vi "LDA_CALCULATOR.vi"() -> ()   [LabVIEW 2013]
uses:
  <vilib>/Utility/file.llb/Read From Spreadsheet File (string).vi
  <vilib>/Utility/file.llb/Read From Spreadsheet File (I64).vi
  <vilib>/Utility/file.llb/Read From Spreadsheet File (DBL).vi
  <vilib>/Analysis/Matrix/Numeric/Conversions/Matrix To Array - RM.vi
  <vilib>/Utility/file.llb/Write To Spreadsheet File (DBL).vi
  <vilib>/Utility/file.llb/Write To Spreadsheet File (I64).vi
  <vilib>/Analysis/Matrix/NI_Matrix.lvlib
panel:
  in  "피험자 이름":path
  in  "SVM_SWLDA_filename":string="SVM_SWLDA_MODEL"
  in  "svm_parameter":T1={"svm_type"=0, "kernel_type"=3, "degree"=3, "gamma"=0.07, "coef0"=0.0, "cache_size"=100.0, "epsilon"=0.001, "C"=1.0, "nr_weight"=0, "weight_label"=[1, 12], "Weight (C(class i))"=[1.0, 1.0], "nu"=0.5, "p"=0.1, "Shrinking"=1, "probability"=1} {"p" format="%.4f"; "nu" format="%.4f"; "Weight (C(class i))" format="%.2f"; "C" format="%.2f"; "epsilon" format="%.4f"; "cache_size" format="%.2f"; "coef0" format="%.2f"; "gamma" format="%.5f"; "kernel_type" items=["Linear", "Poly", "RBF", "Sigmoid"]; "svm_type" items=["C-SVC", "Nu-SVC", "One-class SVM", "epsilon-SVR", "nu-SVR"]}
  in  "SVMfilename":string="SVM_MODEL"
  in  "SWLDA_PREMOVE":dbl=0.1
  in  "SWLDA_PENTER":dbl=0.05
  out "Nontarget_order_array":i64[][](array[numeric])
  out "Target_order_array":i64[](array[numeric])
  out "error out":errorcluster={"status"=TRUE, "code"=10, "source"="Create Folder in Trainging_Set_For_ LDA_Matrix_RSVP.vi<APPEND>\nC:\\Emotion_Research\\_Training_Test(LDA)\\2014-08-30"}
  # "INPUTS"
  # "SWLDA"
  # "SVM"
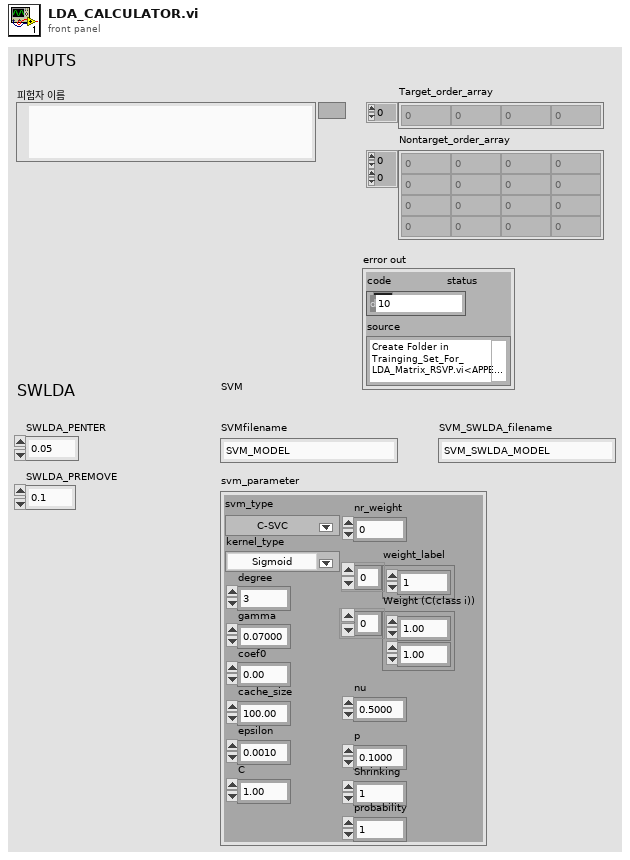
[diagram p1: front panel]
types:
  T1 = cluster{"svm_type":i16, "kernel_type":i16, "degree":i16, "gamma":dbl, "coef0":dbl, "cache_size":dbl, "epsilon":dbl, "C":dbl, "nr_weight":i16, "weight_label":i16[], "Weight (C(class i))":dbl[], "nu":dbl, "p":dbl, "Shrinking":i16, "probability":i16}
  T2 = typedef "NI_Matrix.lvlib/RealMatrix.ctl" = dbl[][]
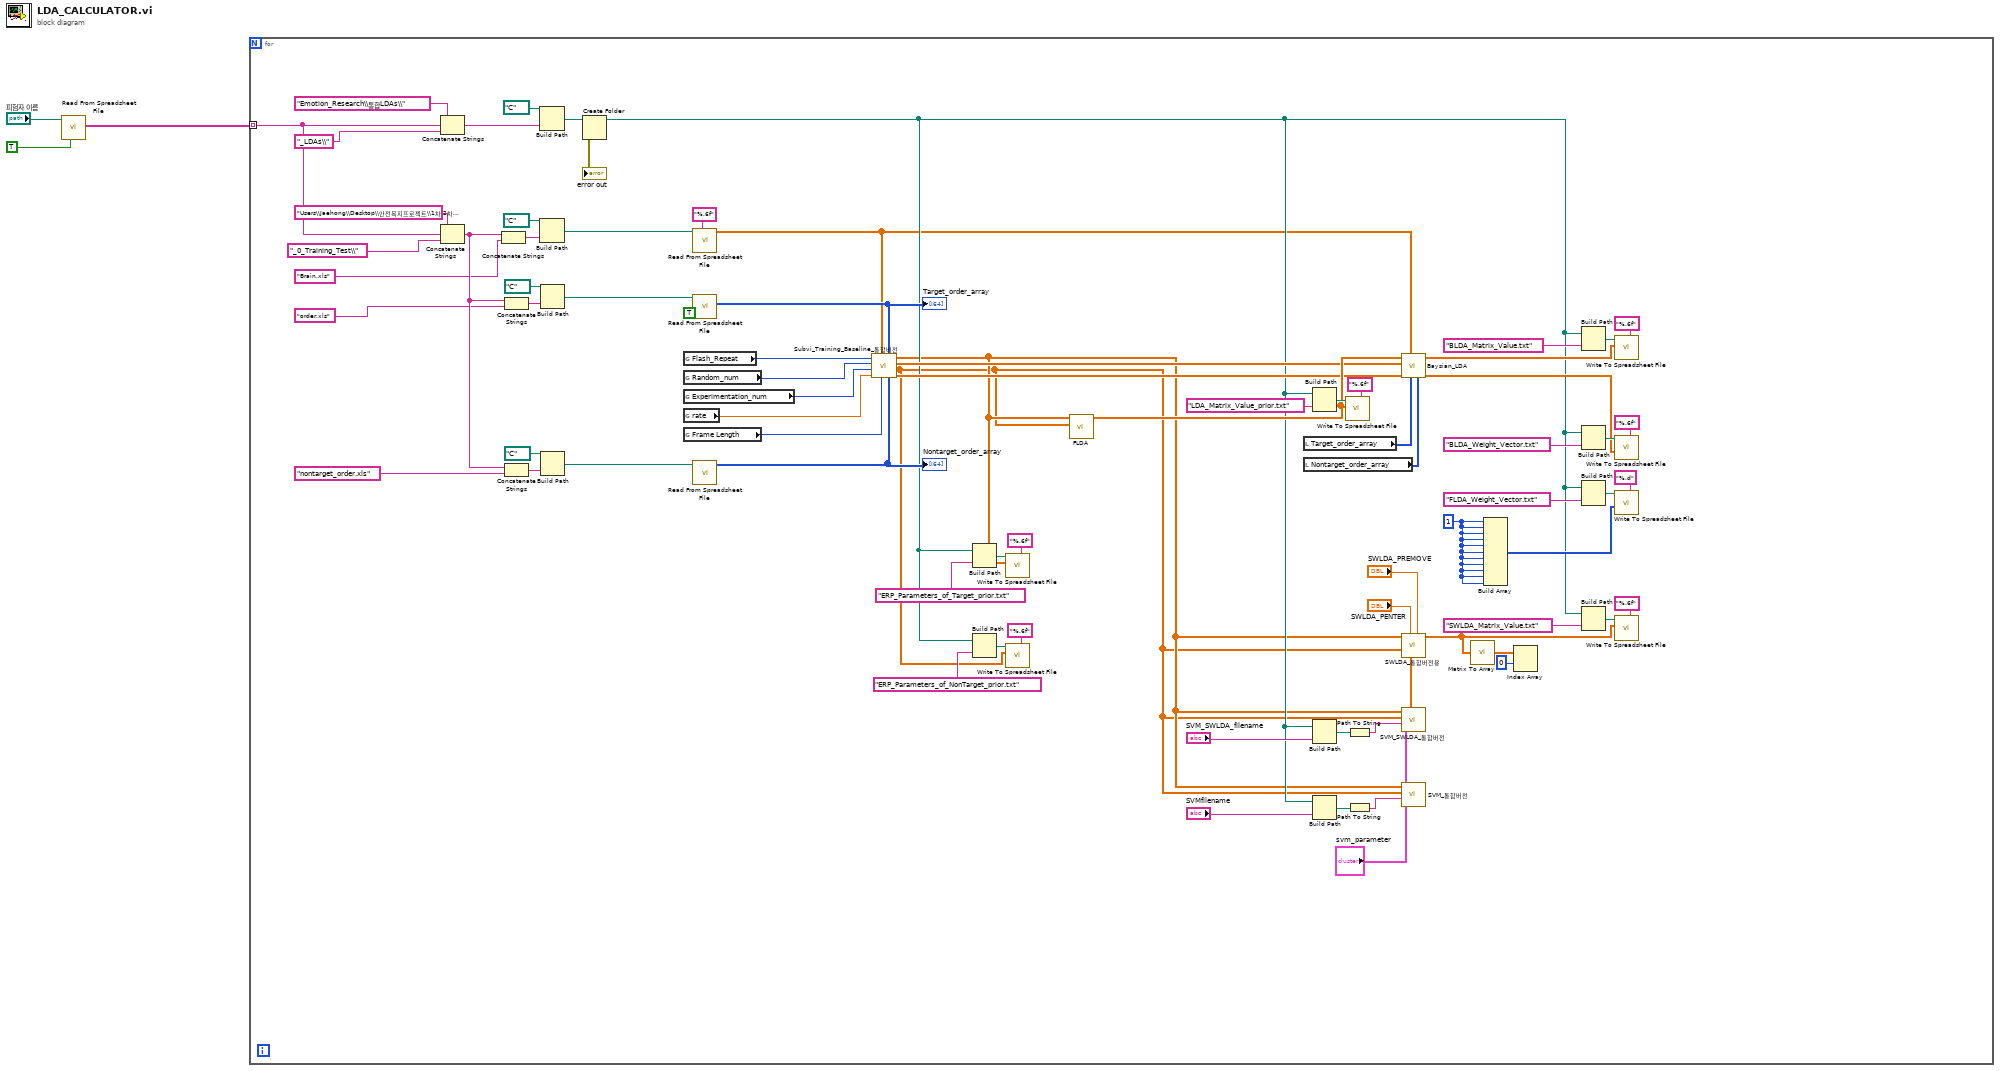
[diagram p0: block diagram]
diagram:
  n1 = call-poly <vilib>:"Read From Spreadsheet File.vi"("transpose (no:F)"=TRUE, "file path (dialog if empty)"="피험자 이름") -> ("first row"=w1:string[])  [unwired: 5 in, 4 out]
  n2 = for {
    tunnel: w1 -> [w18] mode=indexing
    w47 = 1
    n3 = Concatenate Strings("Emotion_Research\\통합LDAs\\" ("string"), w18, "_LDAs\\" ("문자열")) -> (w22:string)
    n4 = Concatenate Strings("Users\\Jaehong\\Desktop\\안전복지프로젝트\\1차 2차 실험 데이터\\Training_Data\\" ("string"), w18, "_0_Training_Test\\" ("문자열")) -> (w15:string)
    n5 = Concatenate Strings(w15, "Brain.xls" ("문자열")) -> (w14:string)
    n6 = Concatenate Strings(w15, "order.xls" ("문자열")) -> (w11:string)
    n7 = Concatenate Strings(w15, "nontarget_order.xls" ("문자열")) -> (w8:string)
    n8 = Build Path(base path=path "C:/" ("path"), name or relative path=w22) -> (appended path=w71:path)
    n9 = Build Path(base path=path "C:/" ("path"), name or relative path=w14) -> (appended path=w12:path)
    n10 = Build Path(base path=path "C:/" ("path"), name or relative path=w11) -> (appended path=w9:path)
    n11 = Build Path(base path=path "C:/" ("path"), name or relative path=w8) -> (appended path=w6:path)
    n12 = Create Folder(path (use dialog)=w71) -> (created path=w28:path, error out=→"error out":errorcluster)  [unwired: 2 in, 1 out]
    n13 = global read "Control_Panel.vi" "Flash_Repeat"() -> (w81:i32)
    n14 = global read "Control_Panel.vi" "Random_num"() -> (w80:i32)
    n15 = global read "Control_Panel.vi" "Experimentation_num"() -> (w79:i32)
    n16 = global read "Control_Panel.vi" "rate"() -> (w78:dbl)
    n17 = global read "Control_Panel.vi" "Frame Length"() -> (w77:i32)
    n18 = call-poly <vilib>:"Read From Spreadsheet File.vi"("format (%.3f)"="%.6f", "file path (dialog if empty)"=w12) -> ("all rows"=w23:dbl[][])  [unwired: 5 in, 4 out]
    n19 = call-poly <vilib>:"Read From Spreadsheet File.vi"("transpose (no:F)"=TRUE, "file path (dialog if empty)"=w9) -> ("first row"=w75:i64[])  [unwired: 5 in, 4 out]
    "Target_order_array" <- w75
    n20 = call-poly <vilib>:"Read From Spreadsheet File.vi"("file path (dialog if empty)"=w6) -> ("all rows"=w74:i64[][])  [unwired: 6 in, 4 out]
    "Nontarget_order_array" <- w74
    n21 = call "Subvi_Training_Baseline_통합버전.vi"("Nontarget_Flash_Order"=w74, "Target_Flash_Order"=w75, "samples per channel"=w77, "Brain_data_source"=w23, "rate"=w78, "Experimentation_num"=w79, "Random_num"=w80, "Random_Repeat"=w81) -> ("Target_ERP"=w33:dbl[][], "NonTarget"=w4:dbl[][], "Nontarget_ERP"=w34:dbl[][], "Target"=w5:dbl[][])
    n22 = Build Path(base path=w28, name or relative path="ERP_Parameters_of_Target_prior.txt") -> (appended path=w66:path)
    n23 = Build Path(base path=w28, name or relative path="ERP_Parameters_of_NonTarget_prior.txt") -> (appended path=w62:path)
    n24 = call-poly <vilib>:"Write To Spreadsheet File.vi"("format (%.3f)"="%.6f", "2D data"=w5, "file path (dialog if empty)"=w66) -> ()  [unwired: 5 in, 1 out]
    n25 = call-poly <vilib>:"Write To Spreadsheet File.vi"("format (%.3f)"="%.6f", "2D data"=w4, "file path (dialog if empty)"=w62) -> ()  [unwired: 5 in, 1 out]
    n26 = call "FLDA.vi"("NonTarget"=w4, "Target"=w5) -> ("A * B 2"=w60:T2)  [unwired: 9 in]
    n27 = local read "Target_order_array"() -> (w57:i64[])
    n28 = local read "Nontarget_order_array"() -> (w56:i64[][])
    n29 = Build Path(base path=w28, name or relative path="LDA_Matrix_Value_prior.txt") -> (appended path=w67:path)
    n30 = Build Path(base path=w28, name or relative path="SVM_SWLDA_filename") -> (appended path=w27:path)
    n31 = Build Path(base path=w28, name or relative path="SVMfilename") -> (appended path=w25:path)
    n32 = call-poly <vilib>:"Write To Spreadsheet File.vi"("format (%.3f)"="%.6f", "2D data"=w60, "file path (dialog if empty)"=w67) -> ()  [unwired: 5 in, 1 out]
    n33 = Path To String(path=w27) -> (string=w26:string)
    n34 = Path To String(path=w25) -> (string=w24:string)
    n35 = call "Baysian_LDA.vi"("nontarget_order"=w56, "target_order"=w57, "RAW__EEG(brain.txt)"=w23, "Target_ERP"=w33, "Nontarget_ERP"=w34, "prior_LDA"=w60) -> ("Weight_vector"=w48:dbl[], "Bayseian_LDA"=w53:T2)  [unwired: 2 in, 2 out]
    n36 = call "SWLDA_통합버전용.vi"("premove"="SWLDA_PREMOVE", "penter"="SWLDA_PENTER", "ERP_Target"=w4, "ERP_Nontarget"=w5) -> ("LDA_matrix"=w37:T2, "WEIGHT"=w31:dbl[])  [unwired: 6 in]
    n37 = call "SVM_SWLDA_통합버전.vi"("WEIGHT"=w31, "svm_parameter"="svm_parameter", "ModelFileName"=w26, "ERP_Parameters_of_Target"=w4, "ERP_Parameters_of_Nontarget"=w5) -> ()  [unwired: 7 in]
    n38 = call "SVM_통합버전.vi"("svm_parameter"="svm_parameter", "ModelFileName"=w24, "ERP_Parameters_of_Target"=w4, "ERP_Parameters_of_Nontarget"=w5) -> ()  [unwired: 8 in]
    n39 = call-poly <vilib>:"Matrix To Array.vi"("Real Matrix"=w37) -> ("Real 2D Array"=w36:dbl[][])
    n40 = Build Array(w47, w47, w47, w47, w47, w47, w47, w47, w47, w47, w47) -> (w43:i32[])
    n41 = Index Array(array=w36, index (row)=0) -> ()  [unwired: 1 in, 1 out]
    n42 = Build Path(base path=w28, name or relative path="BLDA_Matrix_Value.txt") -> (appended path=w54:path)
    n43 = Build Path(base path=w28, name or relative path="BLDA_Weight_Vector.txt") -> (appended path=w51:path)
    n44 = Build Path(base path=w28, name or relative path="FLDA_Weight_Vector.txt") -> (appended path=w45:path)
    n45 = Build Path(base path=w28, name or relative path="SWLDA_Matrix_Value.txt") -> (appended path=w39:path)
    n46 = call-poly <vilib>:"Write To Spreadsheet File.vi"("format (%.3f)"="%.6f", "2D data"=w53, "file path (dialog if empty)"=w54) -> ()  [unwired: 5 in, 1 out]
    n47 = call-poly <vilib>:"Write To Spreadsheet File.vi"("format (%.3f)"="%.6f", "1D data"=w48, "file path (dialog if empty)"=w51) -> ()  [unwired: 5 in, 1 out]
    n48 = call-poly <vilib>:"Write To Spreadsheet File.vi"("format (%d)"="%.d" ("format (%.3f)"), "1D data"=w43, "file path (dialog if empty)"=w45) -> ()  [unwired: 5 in, 1 out]
    n49 = call-poly <vilib>:"Write To Spreadsheet File.vi"("format (%.3f)"="%.6f", "2D data"=w37, "file path (dialog if empty)"=w39) -> ()  [unwired: 5 in, 1 out]
  }
